vi "History Read.vi"(4 "error in (no error)":errorcluster, 6 "Container State":T2, 7 "Display State In":T1) -> (0 "error out":errorcluster, 2 "Value":path[](array[path]), 3 "Display State Out":T1)   [LabVIEW 2009, in "HistoryPath.xctl"]
uses:
  HistoryPath.xctl
  <vilib>/_xctls/Container State.ctl
  State.ctl
  <vilib>/_xctls/XControlSupport.lvlib
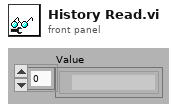
[diagram p1: front panel]
types:
  T1 = typedef "HistoryPath.xctl/State.ctl" = cluster{"History":path[], "History Length":i32}
  T2 = typedef "XControlSupport.lvlib/Container State.ctl" = cluster{"Indicator?":bool, "Run Mode?":bool, " Refnum":refnum<vi>}
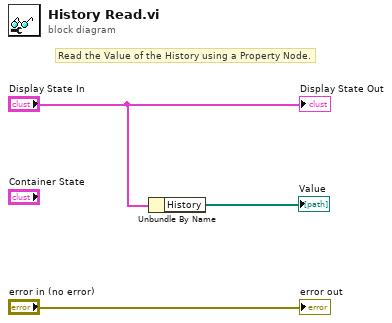
[diagram p0: block diagram]
diagram:
  # "Read the Value of the History using a Property Node."
  n1 = Unbundle By Name("Display State In") -> ("History"=→"Value":path[])
  "error out" <- "error in (no error)"
  "Display State Out" <- "Display State In"
